vi "Add Event.vi"(10 "Event Tag":string, 11 "Item Names in":string[](array[string])) -> (3 "Item Names out":string[](array[string]))   [LabVIEW 2021, in "Game of Life.lvlib"]
uses:
  Game of Life.lvlib
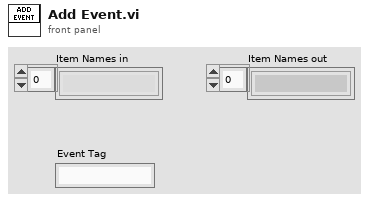
[diagram p1: front panel]
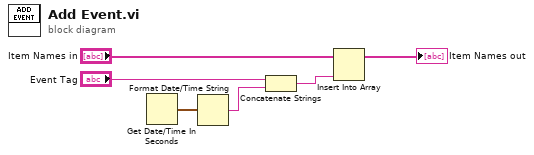
[diagram p0: block diagram]
diagram:
  n1 = Get Date/Time In Seconds() -> (seconds since 1Jan1904=w4:timestamp)
  n2 = Format Date/Time String(seconds (now)=w4) -> (date/time string=w2:string)  [unwired: 2 in]
  n3 = Concatenate Strings("Event Tag", w2) -> (w3:string)
  n4 = Insert Into Array(array="Item Names in", new element=w3) -> (→"Item Names out":string[])  [unwired: 1 in]
